vi "Wait for Request.vi"(8 "error in":errorcluster, 11 "Module in":refnum<class "Module.lvclass">) -> (0 "error out":errorcluster, 1 "Data":variant, 2 "Message":string, 3 "Module out":refnum<class "Module.lvclass">)   [LabVIEW 2020, in "Module.lvlib" / "Module.lvclass"]
uses:
  Module.lvclass
  Module.lvclass/Module.ctl
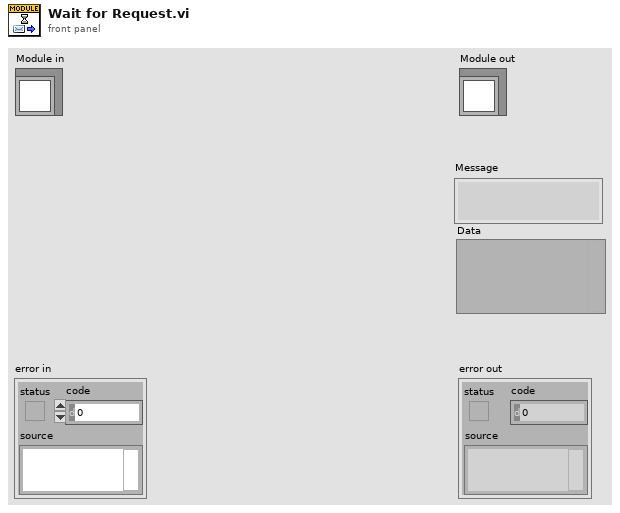
[diagram p1: front panel]
types:
  T1 = typedef "RPC.lvlib/Request.ctl" = cluster{"Method":string, "Params":variant}
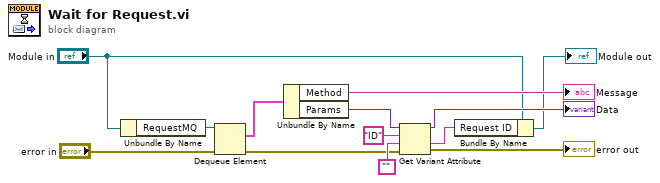
[diagram p0: block diagram]
diagram:
  n1 = Unbundle By Name("Module in") -> ("RequestMQ"=w6:refnum<queue>)
  n2 = Dequeue Element(queue=w6, error in (no error)="error in") -> (element=w9:T1, error out=w7:errorcluster)  [unwired: 1 in, 2 out]
  n3 = Unbundle By Name(w9) -> ("Method"=→"Message":string, "Params"=w4:variant)
  n4 = Get Variant Attribute(Variant=w4, name="ID", default value (empty Variant)="", error in=w7) -> (duplicate Variant=→"Data":variant, value=w10:string, error out=→"error out":errorcluster)  [unwired: 1 out]
  n5 = Bundle By Name(cluster="Module in", "Request ID"=w10) -> (→"Module out":refnum<class "Module.lvclass">)
